vi "Read TCP Config.vi"(8 "error in (no error)":errorcluster, 11 "Modicon PLC in":refnum<class "MB PLC Client.lvclass">) -> (0 "error out":errorcluster, 2 "TCP Config":T1={"IP Address"="", "Port"=0, "Slave ID"=-1, "Timeout"=10000} {"Slave ID" format="%.0x"}, 3 "Modicon PLC out":refnum<class "MB PLC Client.lvclass">)   [LabVIEW 2018, in "MB PLC Client.lvlib" / "MB PLC Client.lvclass"]
uses:
  MB PLC Client.lvclass
  Types/TCP Config_Cluster.ctl
  MB PLC Client.lvclass/MB PLC Client.ctl
  MB PLC Client.lvlib
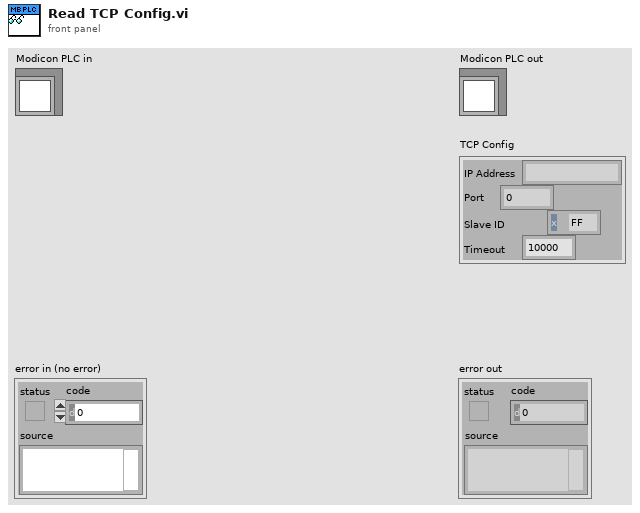
[diagram p1: front panel]
types:
  T1 = typedef "MB PLC Client.lvlib/TCP Config_Cluster.ctl" = cluster{"IP Address":string, "Port":u16, "Slave ID":i8, "Timeout":i32}
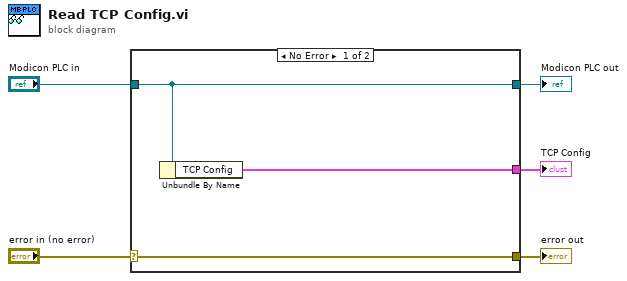
[diagram p0: block diagram]
diagram:
  n1 = case shown="No Error" "error in (no error)" {
    selector: "error in (no error)" -> [w8 w9]
    tunnel: [w8 w9] -> w4
    tunnel: [w7 w10] -> w2
    tunnel: "Modicon PLC in" -> [w7 w10]
    tunnel: [w6 _] -> w1
    frame No Error {
      n2 = Unbundle By Name(w7) -> ("TCP Config"=w6:T1)
    }
    frame Error {
    }
  }
  "error out" <- w4
  "Modicon PLC out" <- w2
  "TCP Config" <- w1
